vi "Main.vi"(11 "Module Admin":refnum<class "Delacor_lib_QMH_Cloneable Module Admin.lvclass">) -> ()   [LabVIEW 2022 SP3, in "ExampleClone.lvlib"]
doc: "This template is based off of the Queued Message Handler design pattern and the Queued Message Handler project template that ships with LabVIEW.\n\nThe main difference is that the queue is private to this module and communication between modules is performed via Broadcast and Request events.\n\nRequest events are wrapped in public API methods and are handled in the Event Handling Loop (EHL) of this VI. Any module can register for Broadcast events sent by this module. The EHL generates messages based on user interface actions.\n\nThe Message Handling Loop (MHL) processes messages generated by the EHL, or by other messages. The messages are string values, so new messages can be added easily to the Message Cases case structure in the MHL. Each message cluster can also provide an optional value for Message Data, which is a variant that can be converted to whatever message-specific data is required.\n____\nHAMPEL SOFTWARE ENGINEERING v2.6.0 (2023-12-19 10:54)"
uses:
  ExampleClone.lvlib
  <vilib>/Delacor/Delacor QMH/Libraries/Cloneable Module Admin_class/Delacor_lib_QMH_Cloneable Module Admin.lvclass
  C:/Program Files/National Instruments/LabVIEW 2022/vi.lib/Delacor/Delacor QMH/Libraries/Module Admin_class/Delacor_lib_QMH_Module Admin.lvclass
  Module Data--cluster.ctl
  <vilib>/Delacor/Delacor QMH/Libraries/Cloneable Module Admin_class/Delacor_lib_QMH_Cloneable Module Admin.lvclass/Delacor_lib_QMH_Cloneable Module Admin.ctl
  Stop Argument--cluster.ctl
  <vilib>/Delacor/Delacor QMH/Libraries/Message Queue_class/Delacor_lib_QMH_Message Queue.lvclass/Delacor_lib_QMH_Message Queue.ctl
  <vilib>/Delacor/Delacor QMH/Libraries/Module Admin_class/Delacor_lib_QMH_Module Admin.lvclass/Delacor_lib_QMH_Module Admin.ctl
  Request UI Display Argument--cluster.ctl
  Libraries/hse-libraries/Source/hse-dqmh/Controls/Module Display Scenarios.ctl
  Request UI Display (Reply Payload)--cluster.ctl
  ExampleMessage Argument--cluster.ctl
  <vilib>/Utility/miscctls.llb/LVPointTypeDef.ctl
  Libraries/hse-libraries/Source/hse-dqmh/Controls/System Message Source.ctl
  <vilib>/Delacor/Delacor QMH/Libraries/Cloneable Module Admin_class/Delacor_lib_QMH_Get Module ID.vi
  <vilib>/Delacor/Delacor QMH/Libraries/Message Queue_class/Delacor_lib_QMH_Enqueue Message (Single).vi
  <vilib>/Delacor/Delacor QMH/Libraries/Module Admin_class/Delacor_lib_QMH_Get External Launch.vi
  <vilib>/Utility/error.llb/Error Cluster From Error Code.vi
  <vilib>/ErrorRing/Error Ring.xnode
  <vilib>/Delacor/Delacor QMH/Libraries/Message Queue_class/Delacor_lib_QMH_Message Queue.lvclass
  Libraries/hse-libraries/Source/hse-dqmh/hse-dqmh.lvlib
panel:
  in  "Btn_SendSystemMessage":bool
  out "Example Message":string
  out "Clone Name":string
  out "Module Name":string
  out "error out":errorcluster
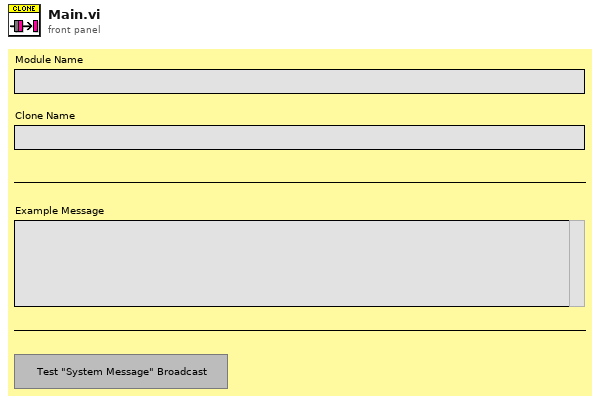
[diagram p1: front panel]
types:
  T1 = typedef "ExampleClone.lvlib/Request Events--cluster.ctl" = cluster{"Stop Module":refnum<user-event>, "Show Panel":refnum<user-event>, "Hide Panel":refnum<user-event>, "Show Diagram":refnum<user-event>, "Get Module Execution Status":refnum<user-event>, "Request UI Display":refnum<user-event>, "Configure":refnum<user-event>, "Prepare":refnum<user-event>, "ExampleMessage":refnum<user-event>}
  T2 = typedef "ExampleClone.lvlib/Module Data--cluster.ctl" = cluster{"Status":string}
  T3 = enum32{"invalid lock state", "Not Locked", "Locked (No Password)", "Password-protected"}
  T4 = typedef "ExampleClone.lvlib/Stop Argument--cluster.ctl" = cluster{"Module ID":i32, "Origin":string, "Exit via Stop Module Req?":bool, "Wait for Module to stop?":bool}
  T5 = typedef "ExampleClone.lvlib/Request UI Display Argument--cluster.ctl" = cluster{"Module ID":i32, "Scenario":T6, "Wait Notifier":refnum<notifier>, "wait for reply":bool}
  T6 = typedef "hse-dqmh.lvlib/Module Display Scenarios.ctl" = enum16{"Stand-Alone", "Managed"}
  T7 = typedef "ExampleClone.lvlib/ExampleMessage Argument--cluster.ctl" = cluster{"Module ID":i32, "ExampleMessage":string}
  T8 = typedef "LVPointTypeDef.ctl" = cluster{"Horizontal":i16, "Vertical":i16}
  T9 = enum32{"Invalid", "Standard", "Closed", "Hidden", "Minimized", "Maximized"}
  T10 = typedef "ExampleClone.lvlib/Request UI Display (Reply Payload)--cluster.ctl" = cluster{"Accept?":bool, "error":errorcluster, "Module ID":i32}
  T11 = typedef "hse-dqmh.lvlib/System Message Source.ctl" = enum16{"module", "application", "network"}
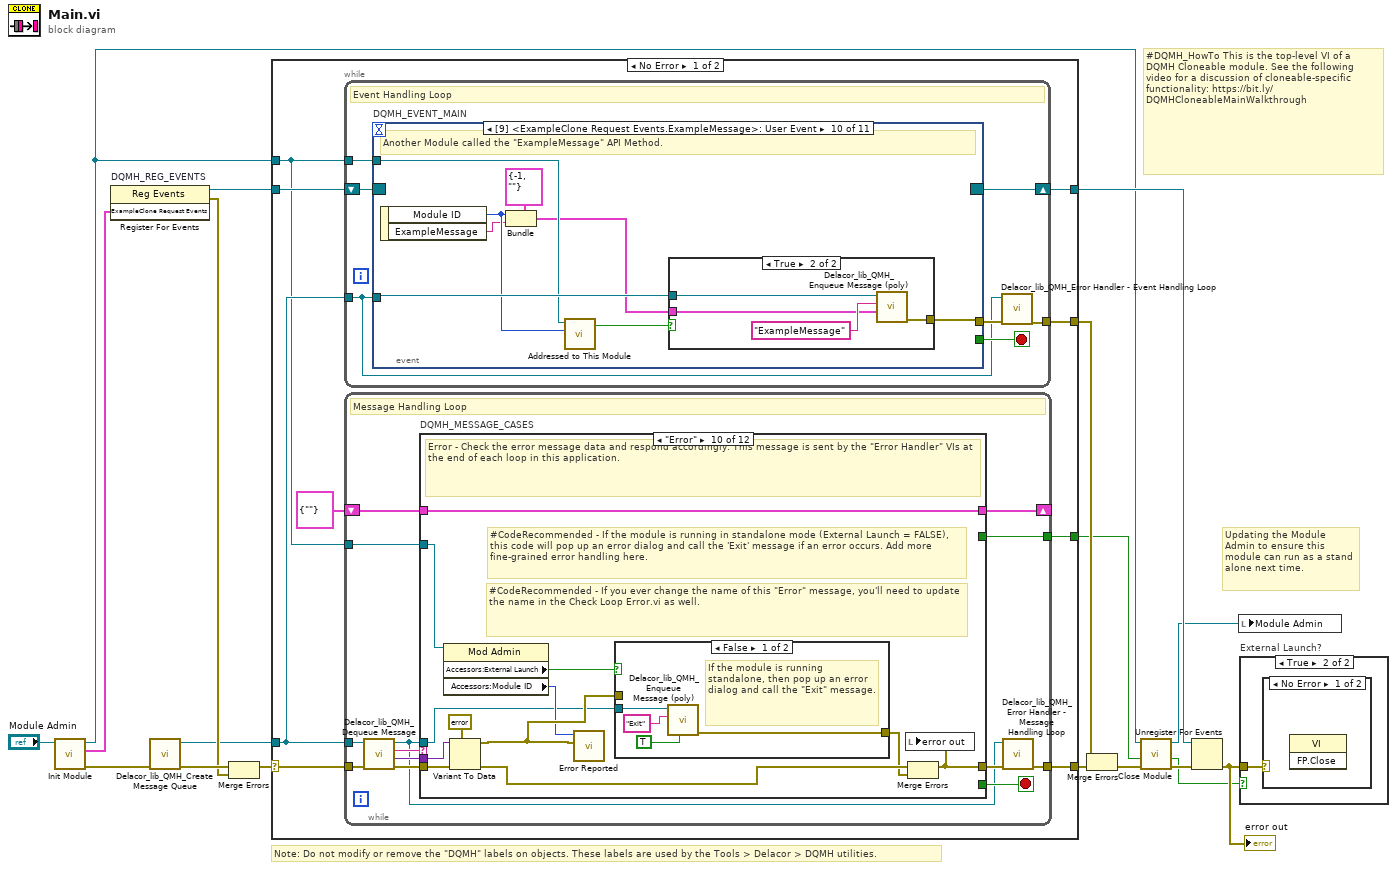
[diagram p0: block diagram]
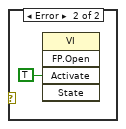
[diagram p3: hidden frame]
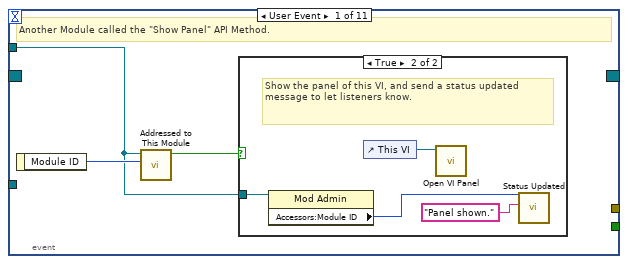
[diagram p4: hidden frame]
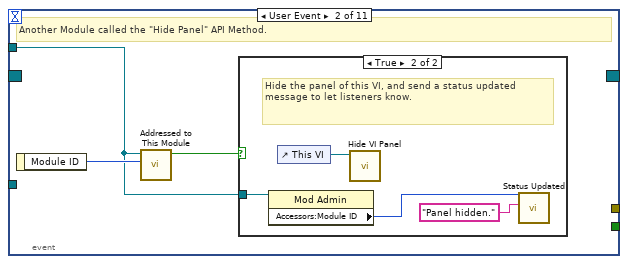
[diagram p6: hidden frame]
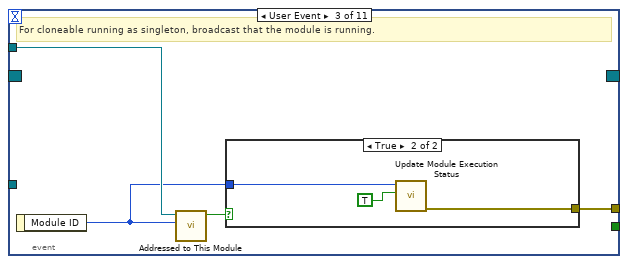
[diagram p8: hidden frame]
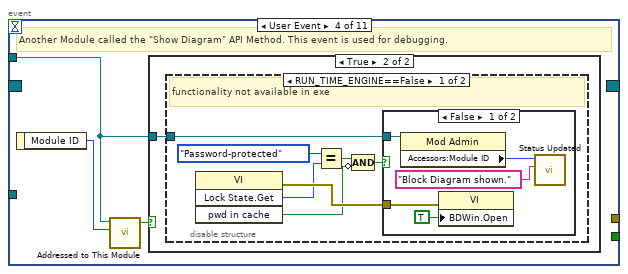
[diagram p10: hidden frame]
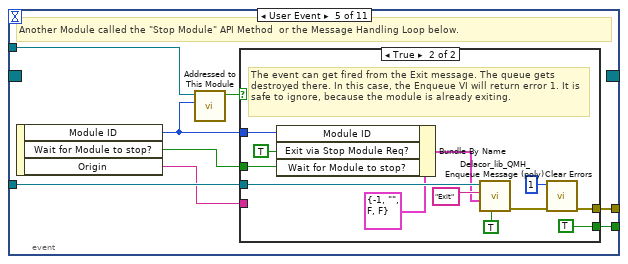
[diagram p14: hidden frame]
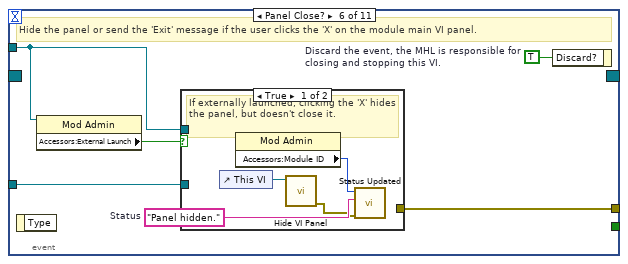
[diagram p16: hidden frame]
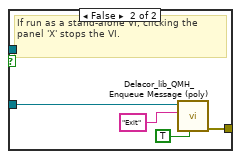
[diagram p17: hidden frame]
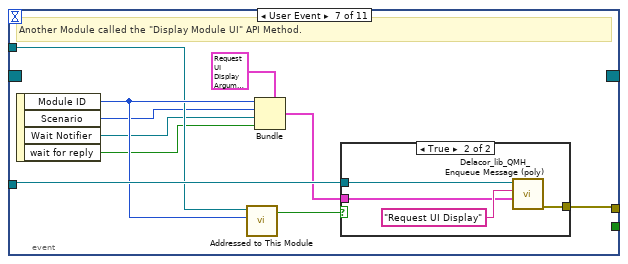
[diagram p18: hidden frame]
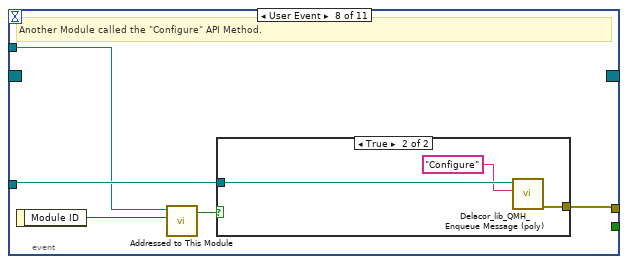
[diagram p20: hidden frame]
diagram:
  # "#DQMH_HowTo This is the top-level VI of a DQMH Cloneable module. See the following video for a discussion of cloneable-specific functionality: https://bit.ly/DQMHCloneableMainWalkthrough"
  # "Note: Do not modify or remove the \"DQMH\" labels on objects. These labels are used by the Tools > Delacor > DQMH utilities."
  # "Updating the Module Admin to ensure this module can run as a stand alone next time."
  n1 = call "Init Module.vi"("Cloneable Module Admin in"="Module Admin") -> ("error out"=w15:errorcluster, "ExampleClone Request Events"=w7:T1, "Cloneable Module Admin out"=w4:refnum<class "Delacor_lib_QMH_Cloneable Module Admin.lvclass">)  [unwired: 8 in]
  n2 = register-events "DQMH_REG_EVENTS"(w7) -> (reference out=w8:refnum<event-registration>, error out=w10:errorcluster)  [unwired: 2 in]
  n3 = call <vilib>:"Delacor_lib_QMH_Create Message Queue.vi"("error in"=w15) -> ("error out"=w12:errorcluster, "Message Queue"=w6:refnum<class "Delacor_lib_QMH_Message Queue.lvclass">)  [unwired: 9 in]
  n4 = Merge Errors(w12, w10) -> (w11:errorcluster)
  n5 = case shown="No Error" w11 {
    selector: w11 -> [w25 w305]
    tunnel: [w27 w305] -> w16
    tunnel: [w24 w314] -> w9
    tunnel: w8 -> [w22 w314]
    tunnel: w6 -> [w21 w307]
    tunnel: [w26 _] -> w17
    tunnel: w4 -> [w20 w310]
    tunnel: [w19 _] -> w2
    frame No Error {
      n6 = while {
        tunnel: w21 -> [w28]
        shift-right: [w31] -> w24
        shift-left: w22 -> [w32]
        tunnel: [w33] -> w26
        tunnel: w20 -> [w29]
        stop <- w30 stop-if-true
        # "Event Handling Loop"
        n7 = event "DQMH_EVENT_MAIN" shown="[9] <ExampleClone Request Events.ExampleMessage>: User Event" {
          selector: w32 -> [_ _ _ _ _ _ _ _ _ _ _]
          dyn-events: [_ _ _ _ _ _ _ _ _ _ _] -> w31
          timeout: _ -> [_ _ _ _ _ _ _ _ _ _ _]
          tunnel: [_ _ _ _ w75 _ _ _ _ _ _] -> w30
          tunnel: w28 -> [_ _ _ _ w78 w94 w115 w124 w132 w143 w150]
          tunnel: [_ _ w52 _ w79 w96 w111 w120 w128 w136 w149] -> w34
          tunnel: w29 -> [w35 w42 w50 w56 w77 w92 w109 w122 w130 w141 _]
          event User Event {
            # "Another Module called the \"Show Panel\" API Method."
            n8 = event-data() -> ("Module ID"=w36:i32)  [unwired: 1 in]
            n9 = call "Addressed to This Module.vi"("Module ID from Argument"=w36, "Module Admin"=w35) -> ("Addressed to this instance?"=w37:bool)  [unwired: 8 in, 1 out]
            n10 = case shown="True" w37 {
              tunnel: w35 -> [_ w39]
              frame False {
              }
              frame True {
                # "Show the panel of this VI, and send a status updated message to let listeners know."
                n11 = property on="Property Node" class="Mod Admin"(reference=w39) -> ("Accessors:Module ID"=w38:i32)  [unwired: 1 in, 2 out]
                n12 = control-ref of="This VI"() -> (w41:refnum<vi>)
                n13 = call "Open VI Panel.vi"("VI"=w41) -> ()  [unwired: 10 in, 1 out]
                n14 = call "Status Updated.vi"("Status"="Panel shown." ("format string"), "Module ID"=w38) -> ()  [unwired: 9 in, 1 out]
              }
            }
          }
          event User Event {
            # "Another Module called the \"Hide Panel\" API Method."
            n15 = event-data() -> ("Module ID"=w43:i32)  [unwired: 1 in]
            n16 = call "Addressed to This Module.vi"("Module ID from Argument"=w43, "Module Admin"=w42) -> ("Addressed to this instance?"=w44:bool)  [unwired: 8 in, 1 out]
            n17 = case shown="True" w44 {
              tunnel: w42 -> [_ w46]
              frame False {
              }
              frame True {
                # "Hide the panel of this VI, and send a status updated message to let listeners know."
                n18 = property on="Property Node" class="Mod Admin"(reference=w46) -> ("Accessors:Module ID"=w45:i32)  [unwired: 1 in, 2 out]
                n19 = control-ref of="This VI"() -> (w48:refnum<vi>)
                n20 = call "Hide VI Panel.vi"("VI"=w48) -> ()  [unwired: 10 in, 1 out]
                n21 = call "Status Updated.vi"("Status"="Panel hidden." ("format string"), "Module ID"=w45) -> ()  [unwired: 9 in, 1 out]
              }
            }
          }
          event User Event {
            # "For cloneable running as singleton, broadcast that the module is running."
            n22 = event-data() -> ("Module ID"=w49:i32)  [unwired: 1 in]
            n23 = call "Addressed to This Module.vi"("Module ID from Argument"=w49, "Module Admin"=w50) -> ("Addressed to this instance?"=w51:bool)  [unwired: 8 in, 1 out]
            n24 = case shown="True" w51 {
              tunnel: [_ w55] -> w52
              tunnel: w49 -> [_ w54]
              frame False {
              }
              frame True {
                n25 = call "Update Module Execution Status.vi"("Running?"=TRUE, "Module ID"=w54) -> ("error out"=w55:errorcluster)  [unwired: 9 in]
              }
            }
          }
          event User Event {
            # "Another Module called the \"Show Diagram\" API Method. This event is used for debugging."
            n26 = event-data() -> ("Module ID"=w57:i32)  [unwired: 1 in]
            n27 = call "Addressed to This Module.vi"("Module ID from Argument"=w57, "Module Admin"=w56) -> ("Addressed to this instance?"=w58:bool)  [unwired: 8 in, 1 out]
            n28 = case shown="True" w58 {
              tunnel: w56 -> [_ w59]
              frame False {
              }
              frame True {
                n29 = disable-structure shown="RUN_TIME_ENGINE==False" {
                  disable-tunnel: w59 -> [w60 _]
                  frame condition #0 (active) {
                    # "functionality not available in exe"
                    n30 = invoke on="Invoke Node" class="VI" method="Lock State.Get"() -> (error out=w66:errorcluster, "Get Lock State"=w65:T3, "pwd in cache"=w62:bool)  [unwired: 4 in, 1 out]
                    n31 = Equal?(x=T3."Password-protected", y=w65) -> (x = y?=w63:bool)
                    n32 = Compound Arithmetic op=AND(w63, invert w62) -> (w61:bool)
                    n33 = case shown="False" w61 {
                      tunnel: w66 -> [w71 _]
                      tunnel: w60 -> [w68 _]
                      frame False {
                        n34 = property on="Property Node" class="Mod Admin"(reference=w68) -> ("Accessors:Module ID"=w67:i32)  [unwired: 1 in, 2 out]
                        n35 = property on="Property Node" class="VI"(error in=w71, "BDWin.Open"=TRUE ("Block Diagram Window:Open")) -> ()  [unwired: 1 in, 2 out]
                        n36 = call "Status Updated.vi"("Status"="Block Diagram shown." ("format string"), "Module ID"=w67) -> ()  [unwired: 9 in, 1 out]
                      }
                      frame True {
                        # "Password-protected VI, and the password is not in the cache. Do not show the diagram."
                      }
                    }
                  }
                  frame condition #1 {
                  }
                }
              }
            }
          }
          event User Event {
            # "Another Module called the \"Stop Module\" API Method  or the Message Handling Loop below."
            n37 = event-data() -> ("Module ID"=w73:i32, "Wait for Module to stop?"=w74:bool, "Origin"=w72:string)  [unwired: 1 in]
            n38 = call "Addressed to This Module.vi"("Module ID from Argument"=w73, "Module Admin"=w77) -> ("Addressed to this instance?"=w76:bool)  [unwired: 8 in, 1 out]
            n39 = case shown="True" w76 {
              tunnel: [_ w90] -> w79
              tunnel: w78 -> [_ w86]
              tunnel: [_ TRUE] -> w75
              tunnel: w74 -> [_ w81]
              tunnel: w73 -> [_ w83]
              tunnel: w72 -> [_ _]
              frame False {
              }
              frame True {
                # "The event can get fired from the Exit message. The queue gets destroyed there. In this case, the Enqueue VI will return error 1. It is safe to ignore, because the module is already exiting."
                n40 = Bundle By Name(cluster=T4 {"Module ID"=-1, "Origin"="", "Exit via Stop Module Req?"=FALSE, "Wait for Module to stop?"=FALSE} ("Stop Argument"), "Module ID"=w83, "Exit via Stop Module Req?"=TRUE, "Wait for Module to stop?"=w81) -> (w80:T4)
                n41 = call-poly <vilib>:"Delacor_lib_QMH_Enqueue Message (poly).vi"("Priority Message? (F)"=TRUE, "Message Data"=w80, "Message"="Exit", "Message Queue in"=w86) -> ("error out"=w91:errorcluster)  [unwired: 6 in, 1 out]
                n42 = call <vilib>:"Clear Errors.vi"("error in (no error)"=w91, "specific error code to clear (0: all)"=1) -> ("error out"=w90:errorcluster)  [unwired: 4 in, 1 out]
              }
            }
          }
          event Panel Close? {
            w95 = TRUE  # Discard the event, the MHL is responsible for closing and stopping this VI.
            # "Hide the panel or send the 'Exit' message if the user clicks the 'X' on the module main VI panel."
            n43 = event-data() -> ()  [unwired: 1 in, 1 out]
            n44 = property on="Property Node" class="Mod Admin"(reference=w92) -> ("Accessors:External Launch"=w93:bool)  [unwired: 1 in, 2 out]
            n45 = case shown="True" w93 {
              tunnel: w94 -> [_ w104]
              tunnel: [_ w105] -> w96
              tunnel: w92 -> [w99 _]
              frame True {
                w100 = "Panel hidden."  # Status
                # "If externally launched, clicking the 'X' hides the panel, but doesn't close it."
                n46 = control-ref of="This VI"() -> (w101:refnum<vi>)
                n47 = property class="Mod Admin"(reference=w99) -> ("Accessors:Module ID"=w98:i32)  [unwired: 1 in, 2 out]
                n48 = call "Hide VI Panel.vi"("VI"=w101) -> ("error out"=w97:errorcluster)  [unwired: 10 in]
                n49 = call "Status Updated.vi"("error in (no error)"=w97, "Status"=w100, "Module ID"=w98) -> ()  [unwired: 8 in, 1 out]
              }
              frame False {
                # "If run as a stand-alone VI, clicking the panel 'X' stops the VI."
                n50 = call-poly <vilib>:"Delacor_lib_QMH_Enqueue Message (poly).vi"("Priority Message? (F)"=TRUE, "Message"="Exit", "Message Queue in"=w104) -> ("error out"=w105:errorcluster)  [unwired: 7 in, 1 out]
              }
            }
            n51 = event-data ("Event Filter Node")("Discard?"=w95) -> ()  [unwired: 1 in, 1 out]
          }
          event User Event {
            # "Another Module called the \"Display Module UI\" API Method."
            n52 = event-data() -> ("Module ID"=w112:i32, "Scenario"=w108:T6, "Wait Notifier"=w107:refnum<notifier>, "wait for reply"=w106:bool)  [unwired: 1 in]
            n53 = call "Addressed to This Module.vi"("Module ID from Argument"=w112, "Module Admin"=w109) -> ("Addressed to this instance?"=w114:bool)  [unwired: 8 in, 1 out]
            n54 = Bundle(cluster=T5 {"Module ID"=-1, "Scenario"=enum."Stand-Alone", "Wait Notifier"=refnum, "wait for reply"=FALSE} ("Display Module UI Argument"), "Module ID"=w112, "Scenario"=w108, "Wait Notifier"=w107, "wait for reply"=w106) -> (w113:T5)
            n55 = case shown="True" w114 {
              tunnel: w115 -> [_ w119]
              tunnel: w113 -> [_ w117]
              tunnel: [_ w116] -> w111
              frame False {
              }
              frame True {
                n56 = call-poly <vilib>:"Delacor_lib_QMH_Enqueue Message (poly).vi"("Message Data"=w117, "Message"="Request UI Display", "Message Queue in"=w119) -> ("error out"=w116:errorcluster)  [unwired: 7 in, 1 out]
              }
            }
          }
          event User Event {
            # "Another Module called the \"Configure\" API Method."
            n57 = event-data() -> ("Module ID"=w121:i32)  [unwired: 1 in]
            n58 = call "Addressed to This Module.vi"("Module ID from Argument"=w121, "Module Admin"=w122) -> ("Addressed to this instance?"=w123:bool)  [unwired: 8 in, 1 out]
            n59 = case shown="True" w123 {
              tunnel: w124 -> [_ w127]
              tunnel: [_ w125] -> w120
              frame False {
              }
              frame True {
                n60 = call-poly <vilib>:"Delacor_lib_QMH_Enqueue Message (poly).vi"("Message"="Configure", "Message Queue in"=w127) -> ("error out"=w125:errorcluster)  [unwired: 8 in, 1 out]
              }
            }
          }
          event User Event {
            # "Another Module called the \"Prepare\" API Method."
            n61 = event-data() -> ("Module ID"=w129:i32)  [unwired: 1 in]
            n62 = call "Addressed to This Module.vi"("Module ID from Argument"=w129, "Module Admin"=w130) -> ("Addressed to this instance?"=w131:bool)  [unwired: 8 in, 1 out]
            n63 = case shown="True" w131 {
              tunnel: w132 -> [_ w135]
              tunnel: [_ w133] -> w128
              frame False {
              }
              frame True {
                n64 = call-poly <vilib>:"Delacor_lib_QMH_Enqueue Message (poly).vi"("Message"="Prepare", "Message Queue in"=w135) -> ("error out"=w133:errorcluster)  [unwired: 8 in, 1 out]
              }
            }
          }
          event User Event {
            # "Another Module called the \"ExampleMessage\" API Method."
            n65 = event-data() -> ("Module ID"=w138:i32, "ExampleMessage"=w137:string)  [unwired: 1 in]
            n66 = Bundle(cluster=T7 {"Module ID"=-1, "ExampleMessage"=""} ("ExampleMessage Argument"), "Module ID"=w138, "ExampleMessage"=w137) -> (w139:T7)
            n67 = call "Addressed to This Module.vi"("Module ID from Argument"=w138, "Module Admin"=w141) -> ("Addressed to this instance?"=w142:bool)  [unwired: 8 in, 1 out]
            n68 = case shown="True" w142 {
              tunnel: w143 -> [_ w147]
              tunnel: w139 -> [_ w145]
              tunnel: [_ w144] -> w136
              frame False {
              }
              frame True {
                n69 = call-poly <vilib>:"Delacor_lib_QMH_Enqueue Message (poly).vi"("Message Data"=w145, "Message"="ExampleMessage", "Message Queue in"=w147) -> ("error out"=w144:errorcluster)  [unwired: 7 in, 1 out]
              }
            }
          }
          event "Btn_SendSystemMessage": Value Change {
            # "Another Module called the \"ExampleMessage\" API Method."
            n70 = event-data() -> ()  [unwired: 1 in, 1 out]
            n71 = call-poly <vilib>:"Delacor_lib_QMH_Enqueue Message (poly).vi"("Message"="Send System Message", "Message Queue in"=w150) -> ("error out"=w149:errorcluster)  [unwired: 8 in, 1 out]
          }
        }
        n72 = call-dynamic "Delacor_lib_QMH_Error Handler - Event Handling Loop.vi"("error in"=w34, "Message Queue in"=w28) -> ("dup error in"=w33:errorcluster)  [unwired: 8 in, 1 out]
      }
      n73 = while {
        tunnel: w21 -> [w154]
        shift-right: [w158] -> _
        shift-left: T2 {"Status"=""} ("Data Cluster") -> [w159]
        tunnel: w25 -> [w162]
        tunnel: [w160] -> w27
        tunnel: w20 -> [w152]
        tunnel: [w151] -> w19
        stop <- w157 stop-if-true
        # "Message Handling Loop"
        n74 = call-dynamic "Delacor_lib_QMH_Dequeue Message.vi"("error in"=w162, "Message Queue in"=w154) -> ("error out"=w161:errorcluster, "Message Data"=w155:variant, "Message"=w156:string, "Message Queue out"=w153:refnum<class "Delacor_lib_QMH_Message Queue.lvclass">)  [unwired: 6 in]
        n75 = case "DQMH_MESSAGE_CASES" shown="\"Error\"" w156 {
          selector: w156 -> [_ _ _ _ _ _ _ _ _ _ _ w291]
          tunnel: w153 -> [_ _ _ _ _ _ _ _ _ w249 w281 _]
          tunnel: w161 -> [w183 w187 w195 w199 w213 w235 w242 w246 w248 w259 w287 w293]
          tunnel: [w181 w187 w194 w199 w205 w233 w241 w245 w248 w255 w284 w294] -> w163
          tunnel: w159 -> [w174 w186 w197 w200 w212 w234 w243 w244 w247 w254 w280 w292]
          tunnel: [w174 w186 w197 w200 w212 w234 w243 w244 w247 w254 w280 w292] -> w158
          tunnel: [_ _ _ _ _ _ _ _ _ _ w279 _] -> w157
          tunnel: w155 -> [_ _ _ _ w210 w232 _ _ _ w253 w277 _]
          tunnel: w152 -> [w169 _ w196 _ w201 _ w239 _ _ w252 w274 w289]
          tunnel: [_ _ _ _ _ _ _ _ _ _ w275 _] -> w151
          frame "Initialize" {
            # "Initialize - Any operation that needs to be done before the module can receive messages. Synchronize Caller Events.vi will inform Start Module.vi that the module has launched and is ready to receive messages. Module Did Init.vi will broadcast that the module initialized."
            n76 = call "Synchronize Caller Events.vi"("error in (no error)"=w183, "Module Admin"=w169) -> ("error out"=w182:errorcluster, "Module Admin out"=w168:refnum<class "Delacor_lib_QMH_Cloneable Module Admin.lvclass">)  [unwired: 8 in]
            n77 = control-ref of="This VI"() -> (w166:refnum<vi>)
            n78 = property on="Property Node" class="Mod Admin"(reference=w168) -> ("Accessors:Module ID"=w171:i32, "Accessors:External Launch"=w170:bool)  [unwired: 1 in, 2 out]
            n79 = property on="Property Node" class="VI"(reference=w166) -> ("Clone Name"=→"Clone Name":string)  [unwired: 1 in, 2 out]
            n80 = call "Module Name--constant.vi"("Module ID"=w171) -> ("Module Name"=w178:string)  [unwired: 10 in]
            "Module Name" <- w178
            n81 = property on="Property Node" class="VI"("Front Panel.Title"=w178) -> (reference out=w180:refnum<vi>, error out=w185:errorcluster)  [unwired: 2 in]
            n82 = Select(t=T9."Hidden" ("State"), s=w170, f=T9."Standard" ("State")) -> (s? t:f=w175:T9)
            n83 = invoke on="Invoke Node" class="VI" method="FP.Open"(reference=w180, error in=w185, "State"=w175) -> (reference out=w179:refnum<vi>, error out=w184:errorcluster)  [unwired: 2 in, 3 out]
            n84 = call "Module Name--constant.vi"("Module ID"=w171) -> ("Module Name"=w172:string)  [unwired: 10 in]
            n85 = local write "Example Message"("" ("Example Message")) -> ()
            n86 = invoke on="Invoke Node" class="VI" method="FP.Center"(reference=w179, error in=w184) -> ()  [unwired: 1 in, 3 out]
            n87 = property on="Pane" class="Pane"("Origin"=T8 {"Horizontal"=0, "Vertical"=0}) -> ()  [unwired: 2 in, 2 out]
            n88 = call "Module Did Init.vi"("error in (no error)"=w182, "Initialized?"=TRUE, "Origin"=w172, "Module ID"=w171) -> ("error out"=w181:errorcluster)  [unwired: 7 in]
          }
          frame "--- Module Specific ---" {
            # "Separator -- The following cases handle messages specific to this Module."
          }
          frame "Configure" {
            # "don't forget to unregister when\nstopping the module."
            # "Triggers the auto-configuration of the module"
            n89 = property on="Property Node" class="Mod Admin"(reference=w196) -> ("Accessors:Module ID"=w190:i32)  [unwired: 1 in, 2 out]
            n90 = control-ref of="This VI"() -> (w188:refnum<vi>)
            n91 = call "Module Name--constant.vi"("Module ID"=w190) -> ("Module Name"=w189:string)  [unwired: 10 in]
            n92 = property on="Property Node" class="VI"("Front Panel.Title"=w189) -> ()  [unwired: 2 in, 2 out]
            n93 = call "DQMH System Message - Add to Run-Time Menu.vi"("Module Descriptor"=w189, "Main VI Reference"=w188) -> ("Payload"=w192:variant, "Identifier"=w191:string, "Source"=w193:T11)  [unwired: 7 in]
            n94 = call "System Message.vi"("Sys. Msg. Source"=w193, "error in (no error)"=w195, "Payload"=w192, "Identifier"=w191, "Module ID"=w190) -> ("error out"=w194:errorcluster)  [unwired: 6 in]
          }
          frame "Prepare" {
            w198 = ""  # Example Message
            # "Prepares the module UI (front panel) for display"
            n95 = local write "Example Message"(w198) -> ()
          }
          frame "Request UI Display" {
            # "Requests another module to display its UI in the given <b>Display Scenario</b>: The \"Stand-Alone\" scenario asks the module to open its front panel as a new windows. The \"Managed\" scenario asks the module to broadcast a request for display which the UI Manager then processes, showing the module in its subpanel."
            n96 = Variant To Data(error in=w213, type=T5 {"Module ID"=-1, "Scenario"=enum."Stand-Alone", "Wait Notifier"=refnum, "wait for reply"=FALSE} ("Request UI Display Argument"), Variant=w210) -> (data=w208:T5, error out=w211:errorcluster)
            n97 = Unbundle By Name(w208) -> ("Module ID"=w203:i32, "Scenario"=w204:T6, "Wait Notifier"=w207:refnum<notifier>, "wait for reply"=w206:bool)
            n98 = control-ref of="This VI"() -> (w202:refnum<vi>)
            n99 = case shown="\"Managed\"" w204 {
              tunnel: w202 -> [w216 w220]
              tunnel: w203 -> [_ w221]
              tunnel: [w215 w222] -> w214
              frame "Stand-Alone", Default {
                n100 = call "Open VI Panel.vi"("VI"=w216) -> ("error out"=w215:errorcluster)  [unwired: 10 in]
              }
              frame "Managed" {
                n101 = call "DQMH System Message - Ready for Display.vi"("Main VI Reference"=w220) -> ("Payload"=w217:variant, "Identifier"=w218:string, "Source"=w219:T11)  [unwired: 8 in]
                n102 = call "System Message.vi"("Sys. Msg. Source"=w219, "Payload"=w217, "Identifier"=w218, "Module ID"=w221) -> ("error out"=w222:errorcluster)  [unwired: 7 in]
              }
            }
            n103 = case shown="True" w206 {
              tunnel: w207 -> [_ w228]
              tunnel: w214 -> [_ w225]
              tunnel: w201 -> [_ w223]
              frame False {
              }
              frame True {
                n104 = property class="Mod Admin"(reference=w223) -> ("Accessors:Module ID"=w224:i32)  [unwired: 1 in, 2 out]
                n105 = Bundle By Name(cluster=T10 {"Accept?"=FALSE, "error"={"status"=FALSE, "code"=0, "source"=""}, "Module ID"=0} ("Request UI Display (Reply Payload)"), "error"=w225, "Module ID"=w224) -> (w226:T10)
                n106 = Send Notification(notification=w226, notifier=w228) -> ()  [unwired: 1 in, 2 out]
              }
            }
            n107 = Merge Errors(w211, w214) -> (w205:errorcluster)
          }
          frame "ExampleMessage" {
            # "Send a message to the module that is displayed on its front panel"
            n108 = Variant To Data(error in=w235, type=T7 {"Module ID"=-1, "ExampleMessage"=""} ("ExampleMessage Argument"), Variant=w232) -> (data=w230:T7, error out=w233:errorcluster)
            n109 = Unbundle By Name(w230) -> ("ExampleMessage"=→"Example Message":string)
          }
          frame "Send System Message" {
            w236 = variant  # Payload
            w237 = "Test Message"  # Identifier
            w240 = System_Message_Source."module"  # Source
            # "Send a message to the module that is displayed on its front panel"
            n110 = property on="Property Node" class="Mod Admin"(reference=w239) -> ("Accessors:Module ID"=w238:i32)  [unwired: 1 in, 2 out]
            n111 = call "System Message.vi"("Sys. Msg. Source"=w240, "error in (no error)"=w242, "Payload"=w236, "Identifier"=w237, "Module ID"=w238) -> ("error out"=w241:errorcluster)  [unwired: 6 in]
          }
          frame "---Copy This Frame---" {
            # "Duplicate this frame when creating new messages.  Change this comment in the duplicated frame to describe this message."
            n112 = Merge Errors(w246) -> (w245:errorcluster)
          }
          frame "--- Exit and Error Handling---" {
            # "Separator - the following cases handle errors and exit messages."
          }
          frame "Error" {
            # "#CodeRecommended - If you ever change the name of this \"Error\" message, you'll need to update the name in the Check Loop Error.vi as well."
            # "#CodeRecommended - If the module is running in standalone mode (External Launch = FALSE), this code will pop up an error dialog and call the 'Exit' message if an error occurs. Add more fine-grained error handling here."
            # "Error - Check the error message data and respond accordingly. This message is sent by the \"Error Handler\" VIs at the end of each loop in this application."
            n113 = property on="Property Node" class="Mod Admin"(reference=w252) -> ("Accessors:External Launch"=w250:bool, "Accessors:Module ID"=w251:i32)  [unwired: 1 in, 2 out]
            n114 = Variant To Data(error in=w259, type=errorcluster {"status"=FALSE, "code"=0, "source"=""} ("error constant"), Variant=w253) -> (data=w260:errorcluster, error out=w257:errorcluster)
            n115 = call "Error Reported.vi"("Error"=w260, "Module ID"=w251) -> ()  [unwired: 9 in, 1 out]
            n116 = case shown="False" w250 {
              tunnel: [w264 _] -> w256
              tunnel: w249 -> [w263 _]
              tunnel: w260 -> [_ _]
              frame False {
                # "If the module is running standalone, then pop up an error dialog and call the \"Exit\" message."
                n117 = call-poly <vilib>:"Delacor_lib_QMH_Enqueue Message (poly).vi"("Priority Message? (F)"=TRUE, "Message"="Exit", "Message Queue in"=w263) -> ("error out"=w264:errorcluster)  [unwired: 7 in, 1 out]
              }
              frame True {
                # "If the module was launched externally, calling the Error Reported broadcast VI is the only action performed by the \"Error\" message. The module's caller can then process the error appropriately."
              }
            }
            n118 = Merge Errors(w257, w256) -> (w255:errorcluster)
            n119 = local write "error out"(w255) -> ()
          }
          frame "Exit" {
            w278 = 91  # 91: not all Exit messages will have an argument
            w279 = TRUE  # Stop the VI
            # "Release the message queue reference"
            # "Exit - Exit the application."
            n120 = property on="Property Node" class="Mod Admin"(reference=w274) -> (reference out=w273:refnum<class "Delacor_lib_QMH_Cloneable Module Admin.lvclass">, "Accessors:Module ID"=w267:i32)  [unwired: 1 in, 1 out]
            n121 = Variant To Data(error in=w287, type=T4 {"Module ID"=-1, "Origin"="", "Exit via Stop Module Req?"=FALSE, "Wait for Module to stop?"=FALSE} ("Stop Argument"), Variant=w277) -> (data=w272:T4, error out=w282:errorcluster)
            n122 = call <vilib>:"Clear Errors.vi"("error in (no error)"=w282, "specific error code to clear (0: all)"=w278) -> ("error out"=w286:errorcluster)  [unwired: 4 in, 1 out]
            n123 = control-ref of="This VI"() -> (w266:refnum<vi>)
            n124 = call "DQMH System Message - Remove from Run-Time Menu.vi"("Main VI Reference"=w266) -> ("Payload"=w270:variant, "Identifier"=w269:string, "Source"=w268:T11)  [unwired: 8 in]
            n125 = call "Handle Exit.vi"("Stop Argument"=w272, "Module Admin in"=w273, "VI reference"=w266) -> ("error out"=w283:errorcluster, "Wait for Stop?"=w275:bool)  [unwired: 7 in]
            n126 = call-dynamic "Delacor_lib_QMH_Release Message Queue.vi"("error in"=w286, "Message Queue"=w281) -> ("error out"=w285:errorcluster)  [unwired: 9 in]
            n127 = call "System Message.vi"("Sys. Msg. Source"=w268, "Payload"=w270, "Identifier"=w269, "Module ID"=w267) -> ("error out"=w271:errorcluster)  [unwired: 7 in]
            n128 = property class="Mod Admin"(reference=w273) -> ("Accessors:Module ID"=w265:i32)  [unwired: 1 in, 2 out]
            n129 = Merge Errors(w285, w283, w271) -> (w284:errorcluster)
            n130 = call "Error Reported.vi"("Error"=w284, "Module ID"=w265) -> ()  [unwired: 9 in, 1 out]
          }
          frame Default {
            # "'Default' case only runs if there is a message that isn't defined in any of the other cases.  Output a programming error."
            n131 = property on="Property Node" class="Mod Admin"(reference=w289) -> ("Accessors:Module ID"=w288:i32)  [unwired: 1 in, 2 out]
            n132 = call "Module Name--constant.vi"("Module ID"=w288) -> ("Module Name"=w290:string)  [unwired: 10 in]
            n133 = xnode "Error Ring"("parameter 0"=w291, "parameter 1"=w290) -> ("error out"=w295:errorcluster)
            n134 = Merge Errors(w293, w295) -> (w294:errorcluster)
          }
        }
        n135 = call-dynamic "Delacor_lib_QMH_Error Handler - Message Handling Loop.vi"("error in"=w163, "Message Queue in"=w153) -> ("dup error in"=w160:errorcluster)  [unwired: 8 in, 1 out]
      }
    }
    frame Error {
      n136 = call "Synchronize Caller Events.vi"("Module Admin"=w310) -> ("error out"=w306:errorcluster, "Module Admin out"=w309:refnum<class "Delacor_lib_QMH_Cloneable Module Admin.lvclass">)  [unwired: 9 in]
      n137 = property on="Property Node" class="Mod Admin"(reference=w309) -> ("Accessors:Module ID"=w308:i32)  [unwired: 1 in, 2 out]
      n138 = call-dynamic "Delacor_lib_QMH_Release Message Queue.vi"("Message Queue"=w307) -> ()  [unwired: 10 in, 1 out]
      n139 = call "Module Name--constant.vi"("Module ID"=w308) -> ("Module Name"=w313:string)  [unwired: 10 in]
      n140 = Merge Errors(w305, w306) -> (w304:errorcluster)
      n141 = Format Into String(format string="An error occurred during initialization. %s is no longer running.", w313) -> (resulting string=w311:string)  [unwired: 2 in, 1 out]
      n142 = call "Error Reported.vi"("Additional Information"=w311, "Error"=w304, "Module ID"=w308) -> ()  [unwired: 8 in, 1 out]
    }
  }
  n143 = Merge Errors(w17, w16) -> (w18:errorcluster)
  n144 = call "Close Module.vi"("error in (no error)"=w18, "Wait for stop?"=w2, "Module Admin in"=w4) -> ("error out"=w14:errorcluster, "External Launch"=w1:bool, "Module Admin out"=w3:refnum<class "Delacor_lib_QMH_Cloneable Module Admin.lvclass">)  [unwired: 6 in]
  n145 = Unregister For Events(event registration refnum=w9, error in=w14) -> (error out=w13:errorcluster)
  "error out" <- w13
  n146 = local write "Module Admin"(w3) -> ()
  n147 = case "External Launch?" shown="True" w1 {
    tunnel: w13 -> [_ w315]
    frame False {
    }
    frame True {
      n148 = case shown="No Error" w315 {
        frame No Error {
          n149 = invoke on="Invoke Node" class="VI" method="FP.Close"() -> ()  [unwired: 3 in, 3 out]
        }
        frame Error {
          n150 = invoke on="Invoke Node" class="VI" method="FP.Open"("Activate"=TRUE ("Activate?")) -> ()  [unwired: 4 in, 5 out]
        }
      }
    }
  }
